vi "OAT Convert Speed Waveform to XY Graph.vi"(0 "waveform speed profile":waveform(dbl)={"t0"=timestamp(0 s since 1904-01-01), "dt"=0.0, "Y"=[]}, 11 "error in (no error)":errorcluster) -> (4 "dup waveform speed profile":waveform(dbl), 6 "speed profile":T1 {"speed [RPM]" format="%.2f"; "time [s]" format="%.2f"}, 8 "pulse/revolution":i32, 10 "rotation direction":u16(ring) items=["CCW", "CW"], 15 "error out":errorcluster)   [LabVIEW 2017, in "SoundVib_TachProcess.lvlib"]
doc: "Converts a waveform speed profile to an XY graph by extracting the information attached to the waveform speed profile."
uses:
  <vilib>/addons/Sound and Vibration/Order Analysis/Tach Process/SoundVib_TachProcess.lvlib
  <vilib>/addons/Sound and Vibration/Order Analysis/Tach Process/SubVIs/speed profile.ctl
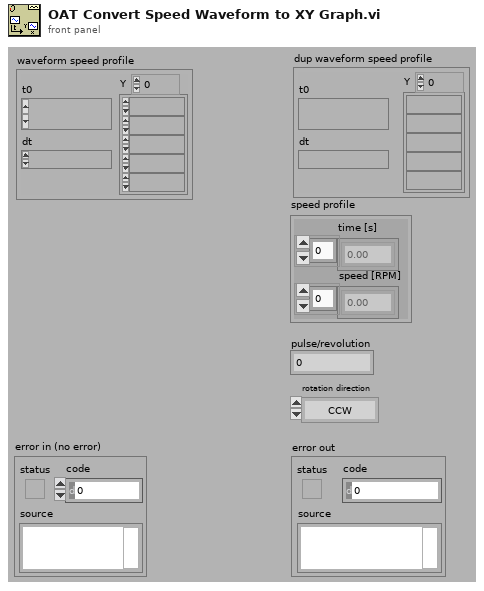
[diagram p1: front panel]
types:
  T1 = typedef "SoundVib_TachProcess.lvlib/speed profile.ctl" = cluster{"time [s]":dbl[], "speed [RPM]":dbl[]}
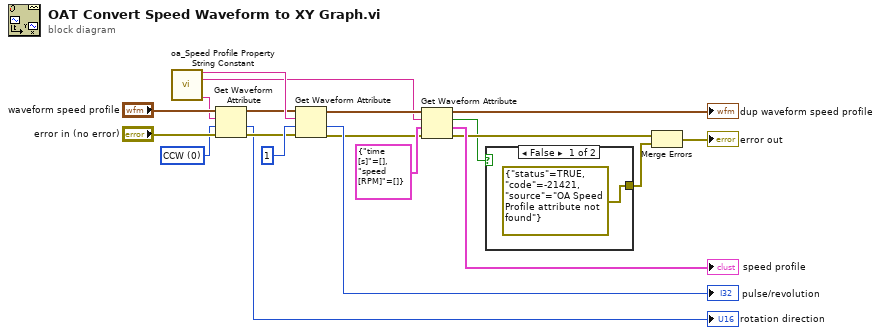
[diagram p0: block diagram]
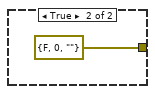
[diagram p2: hidden frame]
diagram:
  w6 = u16 0 items=["CCW", "CW"] ("rotation direction")
  n1 = call <vilib>:"oa_Speed Profile Property String Constant.vi"() -> ("pulse/rev"=w13:string, "speed profile"=w12:string, "rotation direction"=w7:string)  [unwired: 12 in, 1 out]
  n2 = Get Waveform Attribute(4:"error in (no error)", 5:w6, 6:w7, 7:"waveform speed profile") -> (0:w8:errorcluster, 1:→"rotation direction":u16, 3:w9:waveform(dbl))  [unwired: 1 out]
  n3 = Get Waveform Attribute(4:w8, 5:1, 6:w13, 7:w9) -> (0:w15:errorcluster, 1:→"pulse/revolution":i32, 3:w14:waveform(dbl))  [unwired: 1 out]
  n4 = Get Waveform Attribute(4:w15, 5:T1 {"time [s]"=[], "speed [RPM]"=[]} ("speed profile"), 6:w12, 7:w14) -> (0:w4:errorcluster, 1:→"speed profile":T1, 2:w2:bool, 3:→"dup waveform speed profile":waveform(dbl))
  n5 = case shown="False" w2 {
    tunnel: [errorcluster {"status"=TRUE, "code"=-21421, "source"="OA Speed Profile attribute not found"} ("error in") errorcluster {"status"=FALSE, "code"=0, "source"=""} ("error in")] -> w1
    frame False {
    }
    frame True {
    }
  }
  n6 = Merge Errors(w4, w1) -> (→"error out":errorcluster)
